vi "scan result paths.vi"(8 "Error in":errorcluster, 10 "file paths":T1={"Filename profile"=path "C:/Users/microscope/Desktop/Dropbox/RIP/Messungen/SM980_PTP_", "Filename errors"=path "C:/Users/microscope/Desktop/Dropbox/RIP/Messungen/SM980_PTP_Errors_"}, 11 "Action":T2) -> (0 "Error out":errorcluster, 2 "file paths out":T1={"Filename profile"=path "C:/Users/microscope/Desktop/Dropbox/RIP/Messungen/SM980_PTP_", "Filename errors"=path "C:/Users/microscope/Desktop/Dropbox/RIP/Messungen/SM980_PTP_Errors_"})   [LabVIEW 2011]
doc: "Functional Global Variable for the algorithm settings. The used method as well as the max. Iteration steps and the tolerance can be given. In addition, the algorithm can be told to use boundaries (if possible)."
uses:
  Studium/Multilayer University of Bern Folder/controls/FGV_Action.ctl
  controls/scan result path.ctl
panel:
  # "Input"
  # "Output"
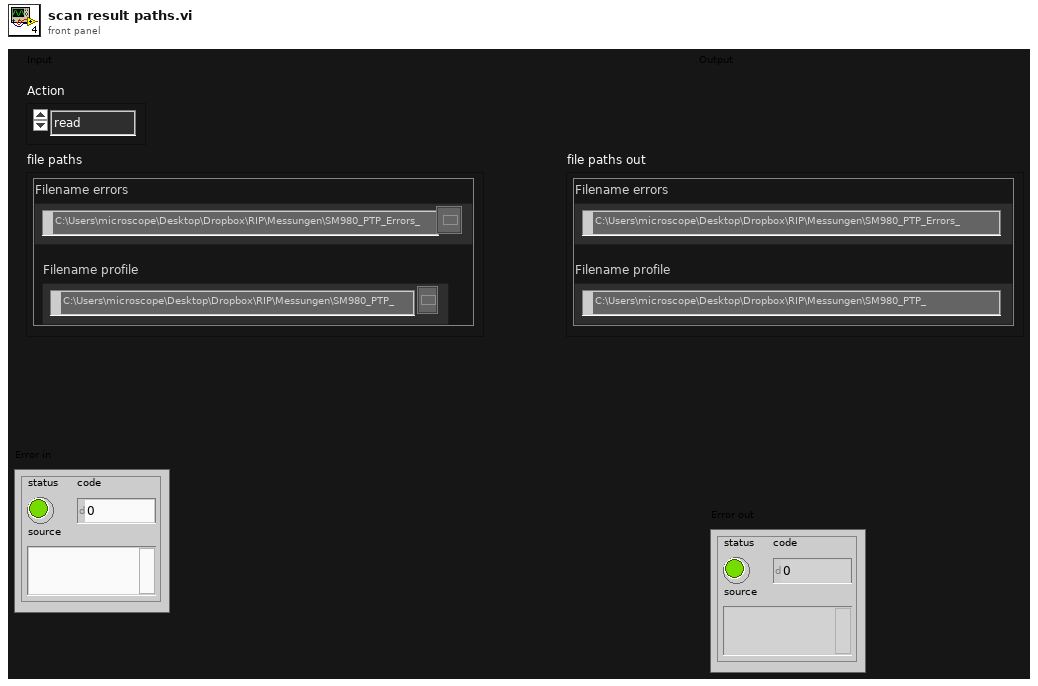
[diagram p1: front panel]
types:
  T1 = typedef "scan result path.ctl" = cluster{"Filename profile":path, "Filename errors":path}
  T2 = typedef "FGV_Action.ctl" = enum16{"read", "write"}
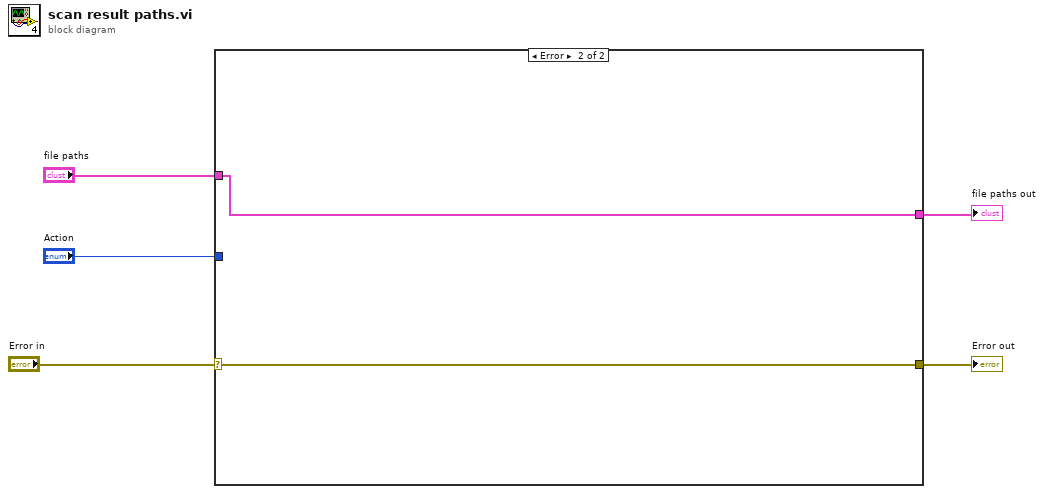
[diagram p0: block diagram]
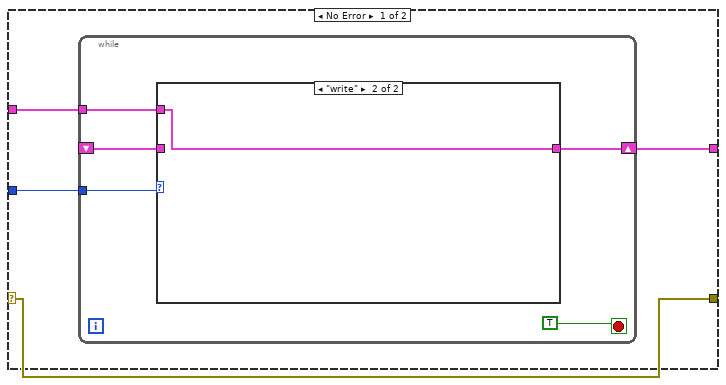
[diagram p2: hidden frame]
diagram:
  n1 = case shown="Error" "Error in" {
    selector: "Error in" -> [w6 w18]
    tunnel: "Action" -> [w9 _]
    tunnel: [w6 w18] -> w4
    tunnel: "file paths" -> [w8 w17]
    tunnel: [w7 w17] -> w2
    frame No Error {
      n2 = while {
        tunnel: w9 -> [w13]
        tunnel: w8 -> [w12]
        shift-right: [w10] -> w7
        shift-left: _ -> [w11]
        stop <- TRUE stop-if-true
        n3 = case shown="\"write\"" w13 {
          tunnel: w12 -> [_ w16]
          tunnel: w11 -> [w15 _]
          tunnel: [w15 w16] -> w10
          frame "read", Default {
          }
          frame "write" {
          }
        }
      }
    }
    frame Error {
    }
  }
  "Error out" <- w4
  "file paths out" <- w2
